vi "Test Override Inherited Test Name.vi"(8 "error in (no error)":errorcluster, 11 "Test Case In":refnum<class "Test Case Test.lvclass">) -> (0 "error out":errorcluster, 3 "Test Case Out":refnum<class "Test Case Test.lvclass">)   [LabVIEW 2020, in "Test Case Test.lvclass"]
uses:
  Test Case Test.lvclass
  C:/Program Files (x86)/National Instruments/LabVIEW 2020/vi.lib/Astemes/LUnit/Test Case.lvclass
  source/Core/Result/Status.ctl
  source/Core/Result/Type.ctl
  <vilib>/Astemes/LUnit/Test Case.lvclass/Test Case.ctl
  <vilib>/Astemes/LUnit/Append Fail Result.vi
  <vilib>/Astemes/LUnit/Append Pass Result.vi
  source/API/LUnit Test Suite/LUnit Test Suite.lvclass
  C:/git/astemes-lunit/source/Core/Runnable/Runnable.lvclass
  Test Case Test.lvclass/Test Case Test.ctl
  Test Doubles/Test Case Test Double Child with Override/Test Case Test Double Child with Override.lvclass
  source/Core/Runnable/Runnable.lvclass
  source/Core/Result/Result.lvlib
  <vilib>/Astemes/LUnit/Test Case.lvclass
  C:/git/astemes-lunit/source/API/LUnit Test Suite/LUnit Test Suite.lvclass
  C:/Program Files (x86)/National Instruments/LabVIEW 2020/vi.lib/Astemes/LUnit/LUnit Runnable.lvclass
  C:/git/astemes-lunit/tests/Test Case Test/Test Case Test.lvclass
panel:
  out "Status":T1
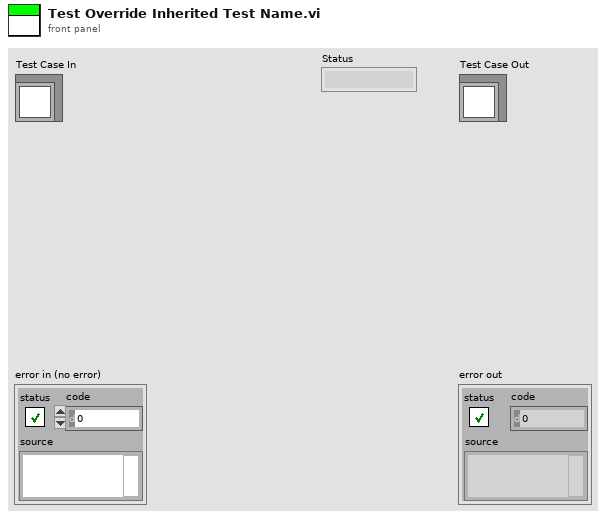
[diagram p1: front panel]
types:
  T1 = typedef "Result.lvlib/Status.ctl" = enum16{"", "Passed", "Failed", "Error", "Skipped", "Setup Error", "Broken", "Teardown Error"}
  T2 = typedef "Result.lvlib/Result.ctl" = cluster{"Name":string, "Message":string, "Description":string, "Status":T1, "Result Type":T3, "Execution Time":dbl}
  T3 = typedef "Result.lvlib/Type.ctl" = enum16{"Test Case", "Test Suite", "Test Run", "Pass", "Fail", "Skip", "Pass if", "Fail if", "Pass if Error", "Fail if Error", "Pass if Equal", "Fail if Equal"}
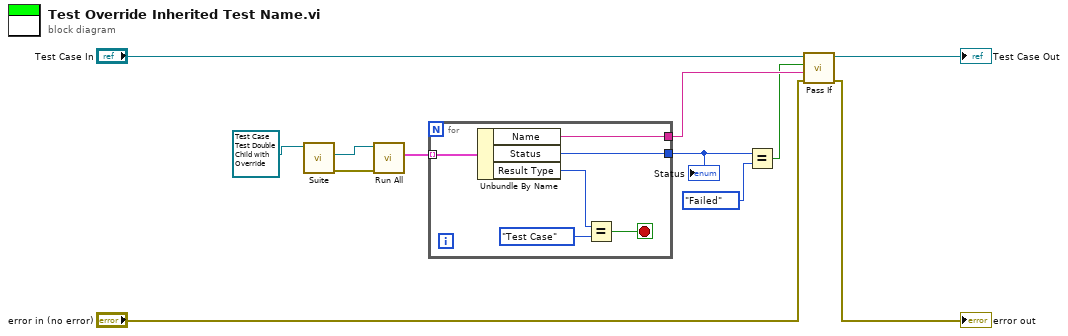
[diagram p0: block diagram]
diagram:
  n1 = call-dynamic "Suite.vi"("LUnit Test Case in"=refnum<class "Test Case Test Double Child with Override.lvclass"> refnum ("Test Case Test Double Child with Override.lvclass")) -> ("error out"=w7:errorcluster, "LUnit Test Suite Out"=w1:refnum<class "LUnit Test Suite.lvclass">)  [unwired: 8 in, 1 out]
  n2 = call "Run All.vi"("error in (no error)"=w7, "Runnable In"=w1) -> ("Results"=w6:T2[])  [unwired: 8 in, 1 out]
  n3 = for {
    tunnel: w6 -> [w18] mode=indexing
    tunnel: [w14] -> w5
    tunnel: [w13] -> w4
    stop <- w15 stop-if-true
    n4 = Unbundle By Name(w18) -> ("Name"=w14:string, "Status"=w13:T1, "Result Type"=w17:T3)
    n5 = Equal?(x=w17, y=Type."Test Case") -> (x = y?=w15:bool)
  }
  "Status" <- w4
  n6 = Equal?(x=w4, y=Status."Failed") -> (x = y?=w2:bool)
  n7 = call <vilib>:"Pass If.vi"("error in (no error)"="error in (no error)", "Message"=w5, "Pass?"=w2, "LUnit Test Case In"="Test Case In") -> ("error out"=→"error out":errorcluster, "LUnit Test Case Out"=→"Test Case Out":refnum<class "Test Case Test.lvclass">)  [unwired: 6 in]
